vi "UpdateSRCountColors.vi"(8 "Error In":errorcluster, 10 "Color Array":u32[](array[numeric]), 11 "Control Refnums":refnum<vi>[](array[refnum])) -> (0 "Error Out":errorcluster)   [LabVIEW 2017, in "Client.lvlib" / "UI_API.lvlib"]
uses:
  UI_API.lvlib
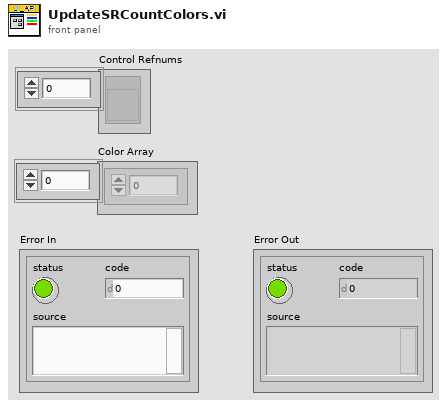
[diagram p1: front panel]
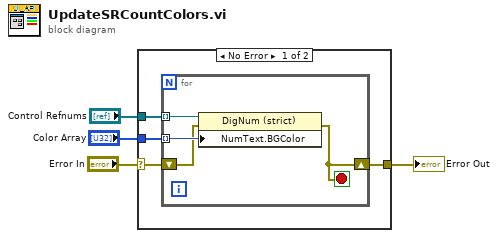
[diagram p0: block diagram]
diagram:
  n1 = case shown="No Error" "Error In" {
    selector: "Error In" -> [w6 w13]
    tunnel: "Control Refnums" -> [w8 _]
    tunnel: "Color Array" -> [w7 _]
    tunnel: [w5 w13] -> w1
    frame No Error {
      n2 = for {
        tunnel: w8 -> [w12] mode=indexing
        tunnel: w7 -> [w11] mode=indexing
        shift-right: [w9] -> w5
        shift-left: w6 -> [w10]
        stop <- w9 stop-if-true
        n3 = property class="DigNum (strict)"(reference=w12, error in=w10, "NumText.BGColor"=w11) -> (error out=w9:errorcluster)  [unwired: 1 out]
      }
    }
    frame Error {
    }
  }
  "Error Out" <- w1
